vi "AuMT8852B Reset Tester.vi"(8 "error in (no error)":errorcluster, 11 "VISA session":refnum<visa-resource-name>) -> (0 "error out":errorcluster, 2 "error code":i32, 3 "VISA session out":refnum<visa-resource-name>)   [LabVIEW 2017]
doc: "Anritsu MT8852B Bluetooth Tester\n\nResets the instrument to a known state. Clears all test results and status information."
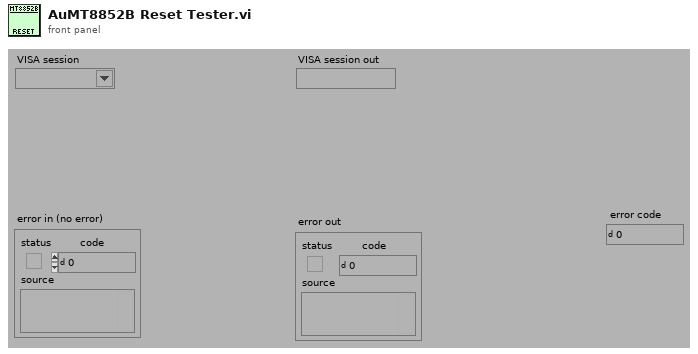
[diagram p1: front panel]
types:
  T1 = enum16{"Simulate", "Range check", "Cache", "Query instrument status"}
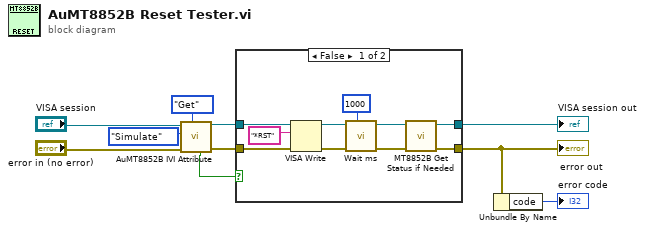
[diagram p0: block diagram]
diagram:
  n1 = call <instrlib>:"AuMT8852B IVI Attribute.vi"("Set/Get (Set)"=enum16{"Set", "Get"}."Get", "error in (no error)"="error in (no error)", "Flag (Simulate)"=T1."Simulate", "VISA session"="VISA session") -> ("error out"=w6:errorcluster, "VISA session out"=w7:refnum<visa-resource-name>, "Value out"=w3:bool)  [unwired: 5 in]
  n2 = case shown="False" w3 {
    tunnel: [w18 w21] -> w10
    tunnel: [w17 w22] -> w1
    tunnel: w7 -> [w20 w21]
    tunnel: w6 -> [w19 w22]
    frame False {
      n3 = VISA Write(VISA resource name=w20, write buffer="*RST" ("write buffer (\"\")"), error in (no error)=w19) -> (VISA resource name out=w14:refnum<visa-resource-name>, error out=w15:errorcluster)  [unwired: 1 out]
      n4 = call <instrlib>:"Wait ms.vi"("Wait (1000 ms)"=u32 1000, "error in (no error)"=w15, "VISA Session"=w14) -> ("error out"=w12:errorcluster, "VISA Session out"=w13:refnum<visa-resource-name>)  [unwired: 7 in]
      n5 = call <instrlib>:"MT8852B Get Status if Needed.vi"("error in (no error)"=w12, "VISA session"=w13) -> ("error out"=w17:errorcluster, "VISA session out"=w18:refnum<visa-resource-name>)  [unwired: 8 in]
    }
    frame True {
    }
  }
  "VISA session out" <- w10
  "error out" <- w1
  n6 = Unbundle By Name(w1) -> ("code"=→"error code":i32)
